vi "Set Application Error from NEC.vi"(8 "Error In":errorcluster, 9 "Log Error?":bool, 10 "Error Source":string, 11 "Error Scope":string) -> (0 "Error Out":errorcluster)   [LabVIEW 2016, in "Stream Error.lvlib" / "Application Error.lvclass"]
doc: "--\nCopyright © 2017 Composed SystemsI All rights reserved.\n\nAuthor: Jon McBee <jon.mcbee@composed.io>\n\nThis library is provided \"AS IS\" ,WITHOUT WARRANTIES OR\nCONDITIONS OF ANY KIND, either express or implied.\n\nComposed Systems -- composed.io\n\nStream 0.0.1.1\nJon McBee - Composed Systems\nCopyright (c) 2017, Composed Systems"
uses:
  <userlib>/Composed Systems/Stream/Error/Classes/Application Error/Application Error.lvclass
  <userlib>/Composed Systems/Stream/Error/Classes/Error Interface/Error Interface.lvclass
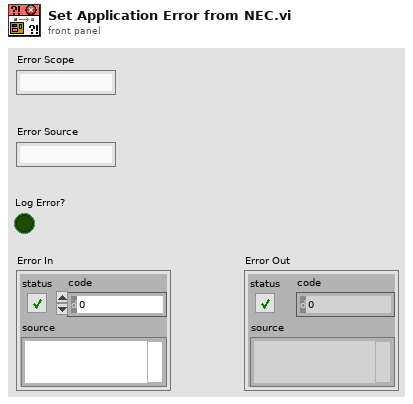
[diagram p1: front panel]
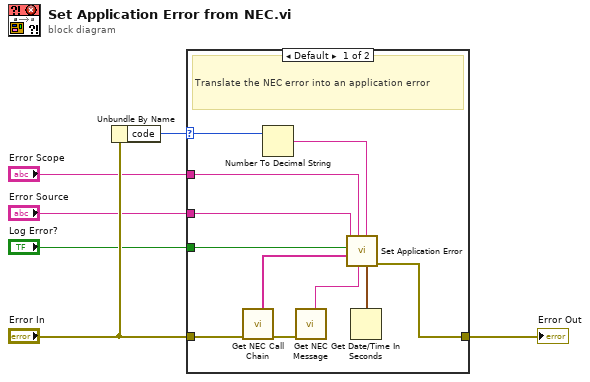
[diagram p0: block diagram]
diagram:
  n1 = Unbundle By Name("Error In") -> ("code"=w5:i32)
  n2 = case shown="Default" w5 {
    selector: w5 -> [w9 _]
    tunnel: "Error In" -> [w17 w18]
    tunnel: [w7 w18] -> w4
    tunnel: "Log Error?" -> [w12 _]
    tunnel: "Error Source" -> [w11 _]
    tunnel: "Error Scope" -> [w10 _]
    frame Default {
      # "Translate the NEC error into an application error"
      n3 = call <userlib>:"Get NEC Call Chain.vi"("error in (no error)"=w17) -> ("error out"=w16:errorcluster, "Call Chain"=w13:string[])  [unwired: 9 in]
      n4 = Number To Decimal String(number=w9) -> (decimal integer string=w8:string)  [unwired: 1 in]
      n5 = call <userlib>:"Get NEC Message.vi"("error in (no error)"=w16) -> ("Message"=w14:string)  [unwired: 9 in, 1 out]
      n6 = Get Date/Time In Seconds() -> (seconds since 1Jan1904=w15:timestamp)
      n7 = call <userlib>:"Set Application Error.vi"("Time Stamp"=w15, "Error Name"=w8, "Error Message"=w14, "Error Scope"=w10, "Call Chain"=w13, "Log Error?"=w12, "Error Source"=w11) -> ("Error Out"=w7:errorcluster)  [unwired: 4 in]
    }
    frame 0, 9999 {
      # "This case handles both No Error and Application Error already embedded in NEC"
    }
  }
  "Error Out" <- w4
